vi "Test Monitoring.vi"(8 "error in":errorcluster, 10 "Socket":u32=1000, 11 "SequenceContext":refnum<k7>) -> (0 "Error Out":errorcluster)   [LabVIEW 2021, in "Diagonistics.lvlib"]
doc: "This VI loops until either the Stop button is pressed or the calling TestStand sequence is terminated. The Termination Monitor VI allows this VI to query the TestStand execution for its current status."
uses:
  Diagonistics.lvlib
  Private Controls/States.ctl
  Private Controls/Local Variables.ctl
  b9d3d6a0-d83f-4724-95f0-26a5c939c190.vi
  c566d1ca-d6ea-491b-8af1-a9688caa810a.vi
  <vilib>/addons/TestStand/_TSUtility.llb/TestStand - Get Property Value (String).vi
  <vilib>/addons/TestStand/_TSUtility.llb/TestStand - Get Property Value (Boolean Array).vi
panel:
  out "Messages":string="Note : "
  out "Test Steps":T1
  out "Elapsed Time":string="0  00:01:15" caption="ms"
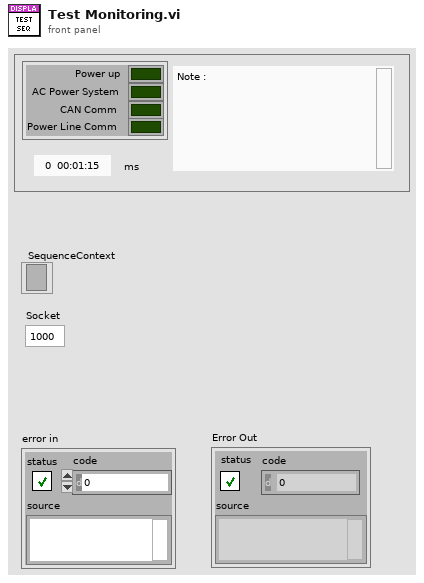
[diagram p1: front panel]
types:
  T1 = cluster{"Power up":bool, "AC Power System":bool, "CAN Comm":bool, "Power Line Comm":bool}
  T2 = typedef "Diagonistics.lvlib/Local Variables.ctl" = cluster{"VI Ref":refnum<vi>, "Messages":refnum<vi>, "Test Steps":refnum<vi>}
  T3 = typedef "Diagonistics.lvlib/States.ctl" = enum16{"Initialization", "Wait for Events", "Exit"}
  T4 = typedef "TestStand - Status Monitor.ctl" = cluster{"Sequence Context":refnum<k7>, "Execution":refnum<k7>, "Termination Monitor":refnum<k7>}
  T5 = cluster{"Value[0]":bool, "Value[1]":bool, "Value[2]":bool, "Value[3]":bool}
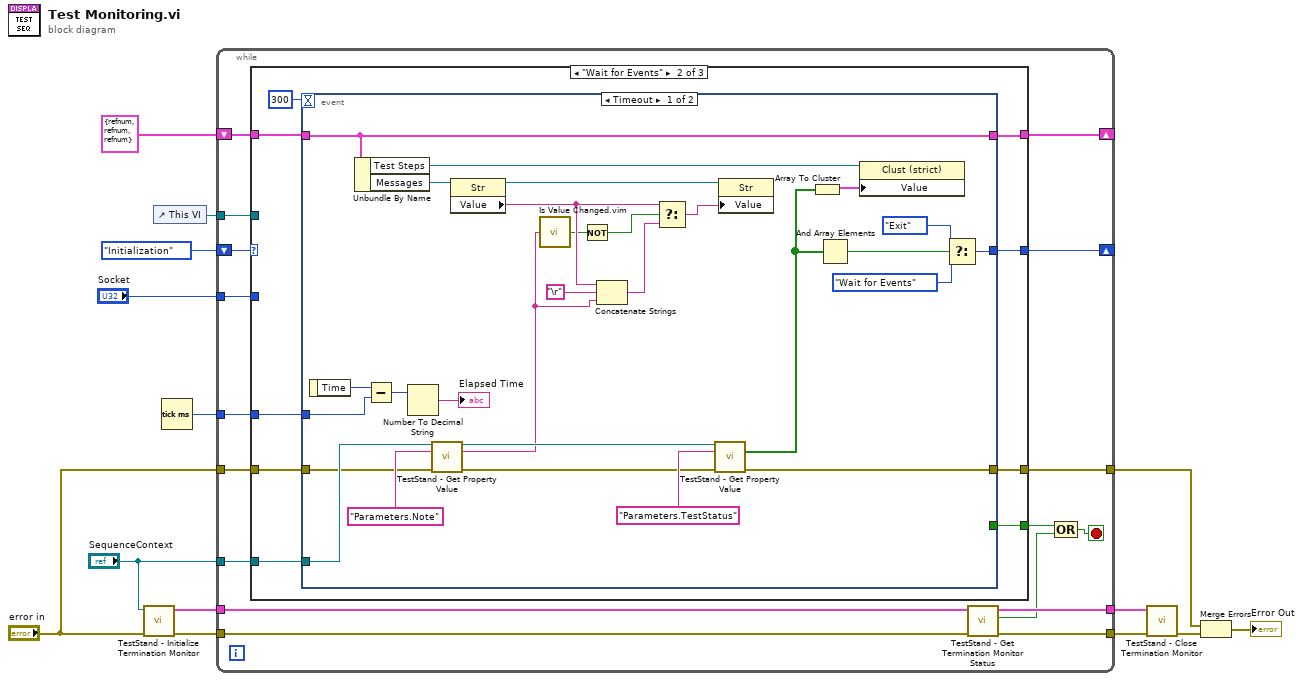
[diagram p0: block diagram]
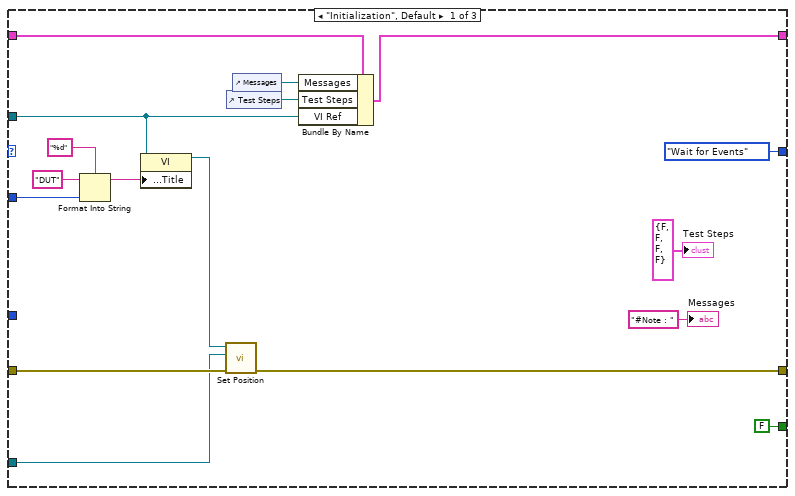
[diagram p2: hidden frame]
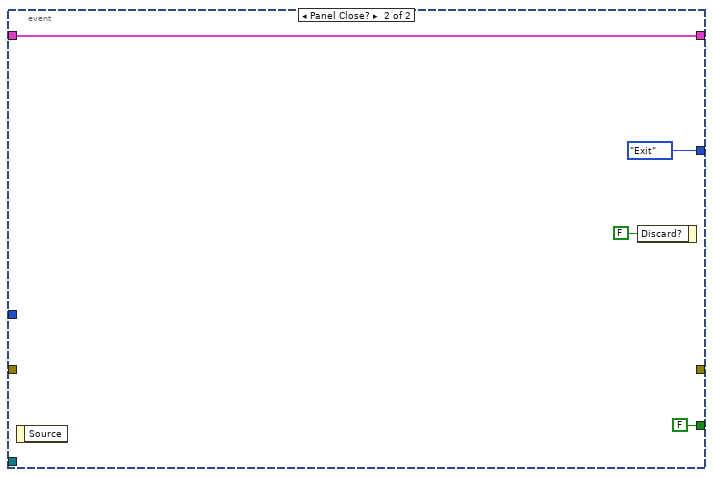
[diagram p3: hidden frame]
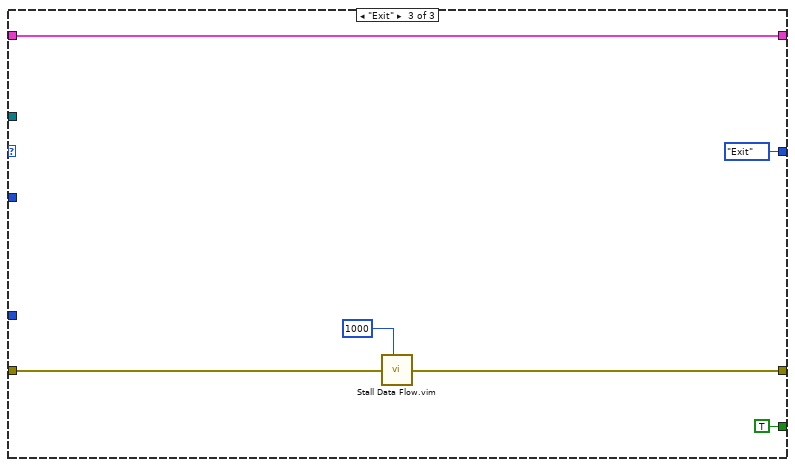
[diagram p4: hidden frame]
diagram:
  n1 = call <vilib>:"TestStand - Initialize Termination Monitor.vi"("error in (no error)"="error in", "Sequence Context In"="SequenceContext") -> ("error out"=w13:errorcluster, "Status Monitor Out"=w12:T4)  [unwired: 8 in]
  n2 = control-ref of="This VI"() -> (w4:refnum<vi>)
  n3 = Tick Count (ms)() -> (millisecond timer value=w5:u32)
  n4 = while {
    tunnel: w12 -> [w31]
    tunnel: [w30] -> w9
    tunnel: w13 -> [w28]
    tunnel: [w22] -> w10
    shift-right: [w23] -> _
    shift-left: T2 {"VI Ref"=refnum, "Messages"=refnum, "Test Steps"=refnum} ("Test Steps") -> [w25]
    tunnel: "SequenceContext" -> [w24]
    shift-right: [w21] -> _
    shift-left: States."Initialization" ("States") -> [w26]
    tunnel: w5 -> [w19]
    tunnel: w4 -> [w18]
    tunnel: "Socket" -> [w17]
    tunnel: "error in" -> [w16]
    tunnel: [w15] -> w2
    stop <- w29 stop-if-true
    n5 = case shown="\"Wait for Events\"" w26 {
      tunnel: w25 -> [w48 w57 w93]
      tunnel: w24 -> [w41 w49 _]
      tunnel: [w47 w53 w93] -> w23
      tunnel: [States."Wait for Events" ("States") w55 States."Exit" ("States")] -> w21
      tunnel: [FALSE ("value") w54 TRUE ("value")] -> w20
      tunnel: w19 -> [_ w52 _]
      tunnel: w18 -> [w45 _ _]
      tunnel: w17 -> [w39 _ _]
      tunnel: w16 -> [w43 w51 w92]
      tunnel: [w36 w50 w91] -> w15
      frame "Initialization", Default {
        n6 = Format Into String(format string="%d", initial string="DUT" ("string"), w39) -> (resulting string=w37:string)  [unwired: 1 in, 1 out]
        n7 = property class="VI"(reference=w45, "Front Panel.Title"=w37) -> (reference out=w42:refnum<vi>)  [unwired: 1 in, 1 out]
        n8 = call "Set Position.vi"("error in"=w43, "Sequence Context In"=w41, "VI Ref"=w42) -> ("error out"=w36:errorcluster)  [unwired: 8 in]
        n9 = control-ref of="Test Steps"() -> (w34:refnum<vi>)
        n10 = control-ref of="Messages"() -> (w35:refnum<vi>)
        n11 = Bundle By Name(cluster=w48, "Messages"=w35, "Test Steps"=w34, "VI Ref"=w45) -> (w47:T2)
        "Test Steps" <- T1 {"Power up"=FALSE, "AC Power System"=FALSE, "CAN Comm"=FALSE, "Power Line Comm"=FALSE} ("Test Steps")
        "Messages" <- "#Note : " ("Messages")
      }
      frame "Wait for Events" {
        n12 = event shown="[0] Timeout" {
          selector: _ -> [_ _]
          dyn-events: _ -> [_ _]
          timeout: 300 -> [_ _]
          tunnel: w57 -> [w85 w87]
          tunnel: [w78 States."Exit" ("States")] -> w55
          tunnel: [_ FALSE ("value")] -> w54
          tunnel: [w85 w87] -> w53
          tunnel: w52 -> [w82 _]
          tunnel: w51 -> [w70 _]
          tunnel: [w68 _] -> w50
          tunnel: w49 -> [w71 _]
          event Timeout {
            n13 = event-data() -> ("Time"=w83:u32)  [unwired: 1 in]
            n14 = Unbundle By Name(w85) -> ("Test Steps"=w74:refnum<vi>, "Messages"=w67:refnum<vi>)
            n15 = Subtract(x=w83, y=w82) -> (x-y=w81:u32)
            n16 = Number To Decimal String(number=w81) -> (decimal integer string=→"Elapsed Time":string)  [unwired: 1 in]
            n17 = call-poly <vilib>:"TestStand - Get Property Value.vi"("Sequence Context In"=w71, "Lookup String"="Parameters.Note", "error in (no error)"=w70) -> ("Sequence Context Out"=w65:refnum<k7>, "Value"=w60:string, "error out"=w69:errorcluster)  [unwired: 10 in]
            n18 = property class="Str"(reference=w67) -> (reference out=w66:refnum<vi>, "Value"=w63:string)  [unwired: 1 in, 1 out]
            n19 = call "Is Value Changed.vim"("value"=w60) -> ("changed or first call?"=w59:bool)
            n20 = Not(x=w59) -> (.not. x?=w58:bool)
            n21 = Concatenate Strings(w63, "\r", w60) -> (w61:string)
            n22 = Select(t=w63, s=w58, f=w61) -> (s? t:f=w64:string)
            n23 = call-poly <vilib>:"TestStand - Get Property Value.vi"("Sequence Context In"=w65, "Lookup String"="Parameters.TestStatus", "error in (no error)"=w69) -> ("Value"=w73:bool[], "error out"=w68:errorcluster)  [unwired: 10 in, 1 out]
            n24 = property class="Str"(reference=w66, "Value"=w64) -> ()  [unwired: 1 in, 2 out]
            n25 = Array To Cluster(array=w73) -> (cluster=w76:T5)
            n26 = And Array Elements(Boolean array=w73) -> (logical AND=w75:bool)
            n27 = property class="Clust (strict)"(reference=w74, "Value"=w76) -> ()  [unwired: 1 in, 2 out]
            n28 = Select(t=States."Exit" ("States"), s=w75, f=States."Wait for Events" ("States")) -> (s? t:f=w78:T3)
          }
          event Panel Close? {
            n29 = event-data() -> ()  [unwired: 1 in, 1 out]
            n30 = event-data("Discard?"=FALSE) -> ()  [unwired: 1 in, 1 out]
          }
        }
      }
      frame "Exit" {
        n31 = call "Stall Data Flow.vim"("value in"=w92, "milliseconds to wait"=u32 1000) -> ("value out"=w91:errorcluster)  [unwired: 1 out]
      }
    }
    n32 = call <vilib>:"TestStand - Get Termination Monitor Status.vi"("error in (no error)"=w28, "Status Monitor In"=w31) -> ("error out"=w22:errorcluster, "Terminating or Aborting"=w27:bool, "Status Monitor Out"=w30:T4)  [unwired: 7 in]
    n33 = Compound Arithmetic op=OR(w20, w27) -> (w29:bool)
  }
  n34 = call <vilib>:"TestStand - Close Termination Monitor.vi"("error in (no error)"=w10, "Status Monitor In"=w9) -> ("error out"=w11:errorcluster)  [unwired: 9 in]
  n35 = Merge Errors(w2, w11) -> (→"Error Out":errorcluster)
